vi "test_232.vi"() -> ()   [LabVIEW 2017]
uses:
  <vilib>/Instr/_visa.llb/VISA Configure Serial Port (Instr).vi
panel:
  out "concatenated string":string
  in  "write buffer":string
  out "error out":errorcluster
  in  "write":bool
  in  "baud rate (9600)":u32=9600
  in  "VISA resource name":refnum<visa-resource-name>
  in  "stop":bool
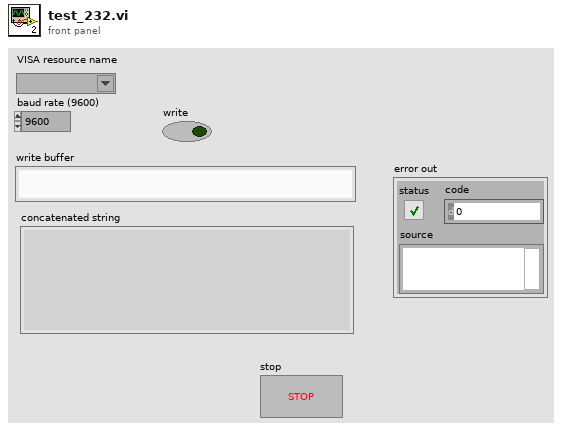
[diagram p1: front panel]
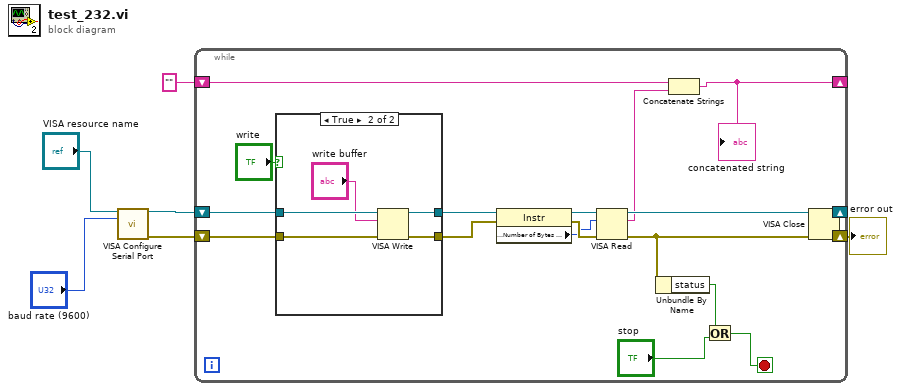
[diagram p0: block diagram]
diagram:
  n1 = call-poly "VISA Configure Serial Port"("VISA resource name"="VISA resource name", "baud rate (9600)"="baud rate (9600)") -> ("VISA resource name out"=w6:refnum<visa-resource-name>, "error out"=w5:errorcluster)  [unwired: 12 in]
  n2 = while {
    shift-right: [w21] -> w8
    shift-left: w6 -> [w20]
    shift-right: [w15] -> w7
    shift-left: w5 -> [w19]
    shift-right: [w9] -> _
    shift-left: "" -> [w10]
    stop <- w12 stop-if-true
    n3 = case shown="True" "write" {
      tunnel: w20 -> [w25 w31]
      tunnel: w19 -> [w26 w30]
      tunnel: [w26 w29] -> w18
      tunnel: [w25 w28] -> w17
      frame False {
      }
      frame True {
        n4 = VISA Write(VISA resource name=w31, write buffer="write buffer", error in (no error)=w30) -> (VISA resource name out=w28:refnum<visa-resource-name>, error out=w29:errorcluster)  [unwired: 1 out]
      }
    }
    n5 = property class="Instr"(reference=w17, error in=w18) -> (reference out=w22:refnum<visa-resource-name>, error out=w24:errorcluster, "Serial Settings:Number of Bytes at Serial Port"=w23:u32)
    n6 = VISA Read(VISA resource name=w22, byte count=w23, error in (no error)=w24) -> (VISA resource name out=w21:refnum<visa-resource-name>, read buffer=w11:string, error out=w15:errorcluster)  [unwired: 1 out]
    n7 = Unbundle By Name(w15) -> ("status"=w13:bool)
    n8 = Concatenate Strings(w10, w11) -> (w9:string)
    "concatenated string" <- w9
    n9 = Or(x=w13, y="stop") -> (x .or. y?=w12:bool)
  }
  n10 = VISA Close(VISA resource name=w8, error in (no error)=w7) -> (error out=→"error out":errorcluster)
